vi "PluginsLoaderCommander_Create.vi"(8 "error in (no error)":errorcluster) -> (0 "error out":errorcluster, 3 "PluginsLoaderCommander out":refnum<class "PluginsLoaderCommander.lvclass">)   [LabVIEW 2014, in "PluginsThread.lvlib" / "PluginsLoaderCommander.lvclass"]
uses:
  PluginsLoaderCommander.lvclass
  PluginsLoaderCommander_CommandData.ctl
  PluginsLoaderCommander_Command.ctl
  PluginsLoaderCommander.lvclass/PluginsLoaderCommander.ctl
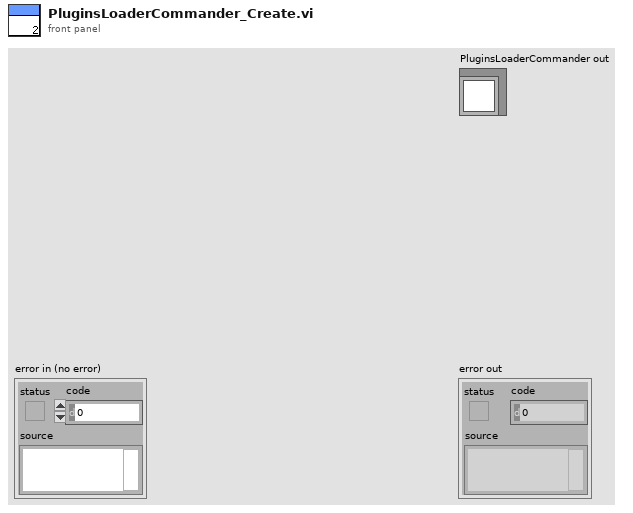
[diagram p1: front panel]
types:
  T1 = typedef "PluginsThread.lvlib/PluginsLoaderCommander.lvclass/PluginsLoaderCommander_CommandData.ctl" = cluster{"Command":T2, "Data":variant}
  T2 = typedef "PluginsThread.lvlib/PluginsLoaderCommander.lvclass/PluginsLoaderCommander_Command.ctl" = enum16{"Stop", "Timeout"}
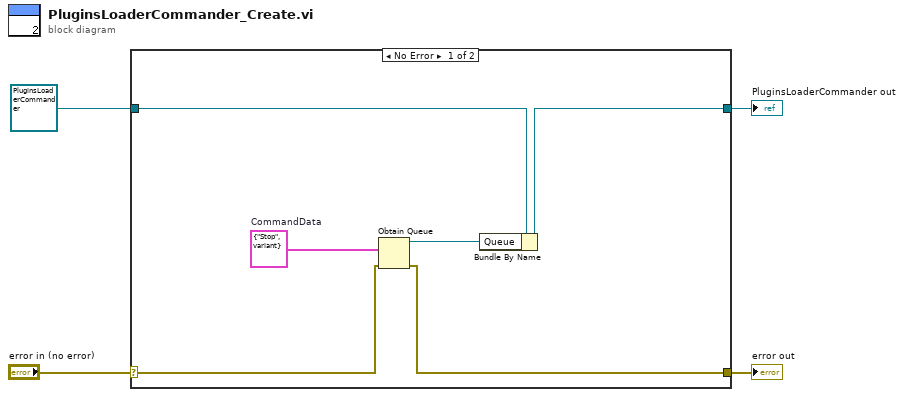
[diagram p0: block diagram]
diagram:
  n1 = case shown="No Error" "error in (no error)" {
    selector: "error in (no error)" -> [w6 w12]
    tunnel: [w5 w12] -> w3
    tunnel: [w8 w11] -> w1
    tunnel: refnum<class "PluginsLoaderCommander.lvclass"> refnum ("PluginsLoaderCommander in") -> [w10 w11]
    frame No Error {
      w9 = T1 {"Command"=enum."Stop", "Data"=variant}  # CommandData
      n2 = Obtain Queue(element data type=w9, error in (no error)=w6) -> (queue out=w7:refnum<queue>, error out=w5:errorcluster)  [unwired: 3 in, 1 out]
      n3 = Bundle By Name(cluster=w10, "Queue"=w7) -> (w8:refnum<class "PluginsLoaderCommander.lvclass">)
    }
    frame Error {
    }
  }
  "error out" <- w3
  "PluginsLoaderCommander out" <- w1
